vi "JLConfig Parse.vi"(0 "Config File Path":path=path "C:/Automation/Configurations/JusticeLeague.ini", 11 "Error In":errorcluster) -> (4 "Pass/Fail?":bool, 6 "Report Text":string, 8 "JusticeLeague_config":T1, 10 "Calibrate":bool, 15 "Error Out":errorcluster)   [LabVIEW 2019]
uses:
  type defs/JLConfig.ctl
  <vilib>/Utility/config.llb/Read Key (String).vi
  <vilib>/Utility/config.llb/Read Key (Boolean).vi
  <vilib>/Utility/config.llb/Read Key (Double).vi
  <vilib>/Utility/config.llb/NI_LVConfig.lvlib
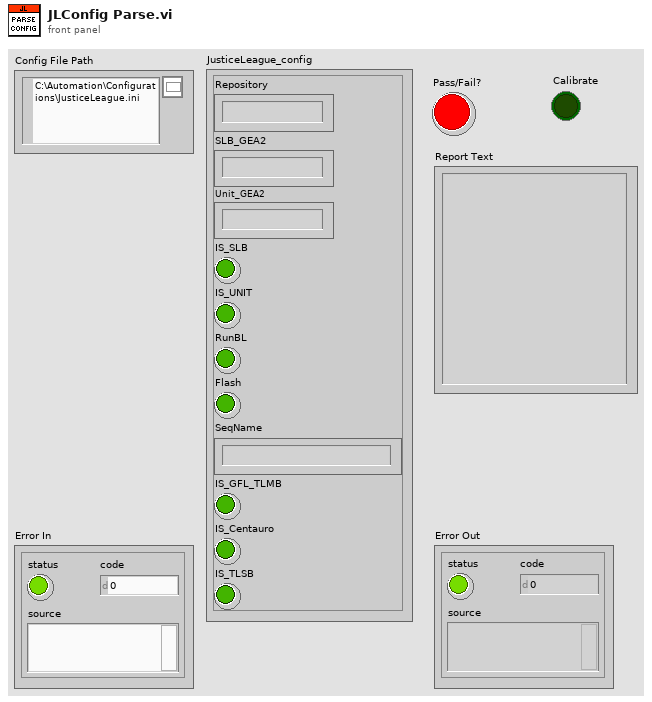
[diagram p1: front panel]
types:
  T1 = typedef "JLConfig.ctl" = cluster{"Repository":string, "SLB_GEA2":string, "Unit_GEA2":string, "IS_SLB":bool, "IS_UNIT":bool, "RunBL":bool, "Flash":bool, "SeqName":string, "IS_GFL_TLMB":bool, "IS_Centauro":bool, "IS_TLSB":bool}
  T2 = cluster{"Calibrate?":bool, "Scalling In ":cluster{"Raw Low ":dbl, "Raw High":dbl, "Actual Low":dbl, "Actual High":dbl}}
  T3 = typedef "NI_LVConfig.lvlib/Config Data RefNum.ctl" = refnum<k1>
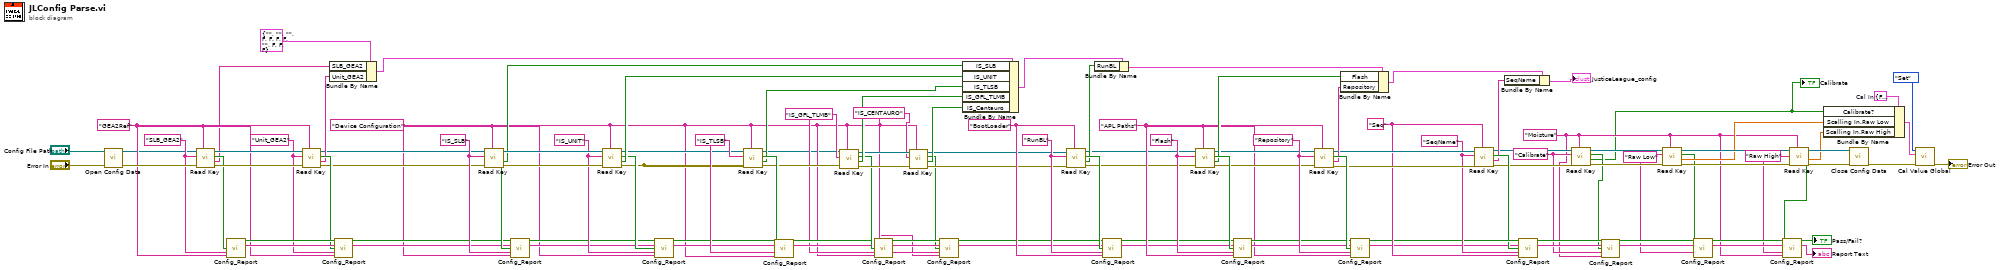
[diagram p0: block diagram]
diagram:
  w14 = "IS_TLSB" ("key")
  w5 = "IS_CENTAURO" ("key")
  w6 = "IS_GFL_TLMB" ("key")
  w34 = "Raw High" ("key")
  w35 = "Raw Low" ("key")
  w51 = T2 {"Calibrate?"=FALSE, "Scalling In "={"Raw Low "=1531.0, "Raw High"=6859.0, "Actual Low"=1.0, "Actual High"=4.9}}  # Cal In
  w33 = "Moisture" ("key")
  w39 = "Calibrate" ("key")
  w65 = "BootLoader" ("key")
  w70 = "RunBL" ("key")
  w83 = "SeqName" ("key")
  w82 = "Seq" ("section")
  w92 = "Repository" ("key")
  w31 = "IS_UNIT" ("key")
  w104 = "Flash" ("key")
  w79 = "APL Paths" ("section")
  w106 = "IS_SLB" ("key")
  w3 = "Device Configuration" ("section")
  w108 = "Unit_GEA2" ("key")
  w113 = "SLB_GEA2" ("key")
  w103 = "GEA2Ref" ("section")
  n1 = call <vilib>:"Open Config Data.vi"("error in (no error)"="Error In", "configuration file path"="Config File Path") -> ("error out"=w116:errorcluster, "refnum"=w86:T3)  [unwired: 7 in, 1 out]
  n2 = call-poly <vilib>:"Read Key.vi"("section"=w103, "error in (no error)"=w116, "key"=w113, "refnum"=w86) -> ("error out"=w117:errorcluster, "value"=w102:string, "found?"=w112:bool, "refnum out"=w118:T3)  [unwired: 4 in]
  n3 = call "Config_Report.vi"("Found?"=w112, "Key"=w113, "Section"=w103) -> ("Pass/Fail"=w111:bool, "Report Text"=w110:string)  [unwired: 11 in]
  n4 = call-poly <vilib>:"Read Key.vi"("section"=w103, "error in (no error)"=w117, "key"=w108, "refnum"=w118) -> ("error out"=w73:errorcluster, "value"=w101:string, "found?"=w109:bool, "refnum out"=w72:T3)  [unwired: 4 in]
  n5 = Bundle By Name(cluster=T1 {"Repository"="", "SLB_GEA2"="", "Unit_GEA2"="", "IS_SLB"=FALSE, "IS_UNIT"=FALSE, "RunBL"=FALSE, "Flash"=FALSE, "SeqName"="", "IS_GFL_TLMB"=FALSE, "IS_Centauro"=FALSE, "IS_TLSB"=FALSE} ("VALEW_config"), "SLB_GEA2"=w102, "Unit_GEA2"=w101) -> (w97:T1)
  n6 = call "Config_Report.vi"("Previous Pass/Fail"=w111, "Previous Report Text"=w110, "Found?"=w109, "Key"=w108, "Section"=w103) -> ("Pass/Fail"=w74:bool, "Report Text"=w75:string)  [unwired: 9 in]
  n7 = call-poly <vilib>:"Read Key.vi"("section"=w3, "error in (no error)"=w73, "key"=w106, "refnum"=w72) -> ("error out"=w99:errorcluster, "value"=w95:bool, "found?"=w107:bool, "refnum out"=w100:T3)  [unwired: 4 in]
  n8 = call "Config_Report.vi"("Previous Pass/Fail"=w74, "Previous Report Text"=w75, "Found?"=w107, "Key"=w106, "Section"=w3) -> ("Pass/Fail"=w29:bool, "Report Text"=w28:string)  [unwired: 9 in]
  n9 = call-poly <vilib>:"Read Key.vi"("section"=w3, "error in (no error)"=w99, "key"=w31, "refnum"=w100) -> ("error out"=w11:errorcluster, "value"=w96:bool, "found?"=w30:bool, "refnum out"=w12:T3)  [unwired: 4 in]
  n10 = call "Config_Report.vi"("Previous Pass/Fail"=w29, "Previous Report Text"=w28, "Found?"=w30, "Key"=w31, "Section"=w3) -> ("Pass/Fail"=w9:bool, "Report Text"=w10:string)  [unwired: 9 in]
  n11 = call-poly <vilib>:"Read Key.vi"("section"=w3, "error in (no error)"=w11, "key"=w14, "refnum"=w12) -> ("value"=w4:bool, "found?"=w13:bool, "refnum out"=w1:T3)  [unwired: 4 in, 1 out]
  n12 = call "Config_Report.vi"("Previous Pass/Fail"=w9, "Previous Report Text"=w10, "Found?"=w13, "Key"=w14, "Section"=w3) -> ("Pass/Fail"=w8:bool, "Report Text"=w7:string)  [unwired: 9 in]
  n13 = call-poly <vilib>:"Read Key.vi"("section"=w3, "error in (no error)"=w11, "key"=w6, "refnum"=w1) -> ("error out"=w19:errorcluster, "value"=w22:bool, "found?"=w16:bool, "refnum out"=w21:T3)  [unwired: 4 in]
  n14 = call "Config_Report.vi"("Previous Pass/Fail"=w8, "Previous Report Text"=w7, "Found?"=w16, "Key"=w6, "Section"=w3) -> ("Pass/Fail"=w26:bool, "Report Text"=w27:string)  [unwired: 9 in]
  n15 = call-poly <vilib>:"Read Key.vi"("section"=w3, "error in (no error)"=w19, "key"=w5, "refnum"=w21) -> ("error out"=w18:errorcluster, "value"=w23:bool, "found?"=w15:bool, "refnum out"=w20:T3)  [unwired: 4 in]
  n16 = call "Config_Report.vi"("Previous Pass/Fail"=w26, "Previous Report Text"=w27, "Found?"=w15, "Key"=w5, "Section"=w3) -> ("Pass/Fail"=w25:bool, "Report Text"=w24:string)  [unwired: 9 in]
  n17 = Bundle By Name(cluster=w97, "IS_SLB"=w95, "IS_UNIT"=w96, "IS_TLSB"=w4, "IS_GFL_TLMB"=w22, "IS_Centauro"=w23) -> (w71:T1)
  n18 = call-poly <vilib>:"Read Key.vi"("section"=w65, "error in (no error)"=w18, "key"=w70, "refnum"=w20) -> ("error out"=w17:errorcluster, "value"=w68:bool, "found?"=w69:bool, "refnum out"=w63:T3)  [unwired: 4 in]
  n19 = Bundle By Name(cluster=w71, "RunBL"=w68) -> (w64:T1)
  n20 = call "Config_Report.vi"("Previous Pass/Fail"=w25, "Previous Report Text"=w24, "Found?"=w69, "Key"=w70, "Section"=w65) -> ("Pass/Fail"=w67:bool, "Report Text"=w66:string)  [unwired: 9 in]
  n21 = call-poly <vilib>:"Read Key.vi"("section"=w79, "error in (no error)"=w17, "key"=w104, "refnum"=w63) -> ("error out"=w88:errorcluster, "value"=w94:bool, "found?"=w105:bool, "refnum out"=w89:T3)  [unwired: 4 in]
  n22 = call "Config_Report.vi"("Previous Pass/Fail"=w67, "Previous Report Text"=w66, "Found?"=w105, "Key"=w104, "Section"=w79) -> ("Pass/Fail"=w91:bool, "Report Text"=w90:string)  [unwired: 9 in]
  n23 = call-poly <vilib>:"Read Key.vi"("section"=w79, "error in (no error)"=w88, "key"=w92, "refnum"=w89) -> ("error out"=w85:errorcluster, "value"=w87:string, "found?"=w93:bool, "refnum out"=w84:T3)  [unwired: 4 in]
  n24 = Bundle By Name(cluster=w64, "Flash"=w94, "Repository"=w87) -> (w78:T1)
  n25 = call "Config_Report.vi"("Previous Pass/Fail"=w91, "Previous Report Text"=w90, "Found?"=w93, "Key"=w92, "Section"=w79) -> ("Pass/Fail"=w81:bool, "Report Text"=w76:string)  [unwired: 9 in]
  n26 = call-poly <vilib>:"Read Key.vi"("section"=w82, "error in (no error)"=w85, "key"=w83, "refnum"=w84) -> ("error out"=w62:errorcluster, "value"=w77:string, "found?"=w80:bool, "refnum out"=w61:T3)  [unwired: 4 in]
  n27 = Bundle By Name(cluster=w78, "SeqName"=w77) -> (→"JusticeLeague_config":T1)
  n28 = call "Config_Report.vi"("Previous Pass/Fail"=w81, "Previous Report Text"=w76, "Found?"=w80, "Key"=w83, "Section"=w82) -> ("Pass/Fail"=w47:bool, "Report Text"=w42:string)  [unwired: 9 in]
  n29 = call-poly <vilib>:"Read Key.vi"("section"=w33, "error in (no error)"=w62, "key"=w39, "refnum"=w61) -> ("error out"=w59:errorcluster, "value"=w32:bool, "found?"=w38:bool, "refnum out"=w60:T3)  [unwired: 4 in]
  "Calibrate" <- w32
  n30 = call "Config_Report.vi"("Previous Pass/Fail"=w47, "Previous Report Text"=w42, "Found?"=w38, "Key"=w39, "Section"=w33) -> ("Pass/Fail"=w46:bool, "Report Text"=w41:string)  [unwired: 9 in]
  n31 = call-poly <vilib>:"Read Key.vi"("section"=w33, "error in (no error)"=w59, "key"=w35, "refnum"=w60) -> ("error out"=w57:errorcluster, "value"=w50:dbl, "found?"=w37:bool, "refnum out"=w58:T3)  [unwired: 4 in]
  n32 = call "Config_Report.vi"("Previous Pass/Fail"=w46, "Previous Report Text"=w41, "Found?"=w37, "Key"=w35) -> ("Pass/Fail"=w45:bool, "Report Text"=w40:string)  [unwired: 10 in]
  n33 = call-poly <vilib>:"Read Key.vi"("section"=w33, "error in (no error)"=w57, "key"=w34, "refnum"=w58) -> ("error out"=w56:errorcluster, "value"=w49:dbl, "found?"=w36:bool, "refnum out"=w55:T3)  [unwired: 4 in]
  n34 = call "Config_Report.vi"("Previous Pass/Fail"=w45, "Previous Report Text"=w40, "Found?"=w36, "Key"=w34, "Section"=w33) -> ("Pass/Fail"=→"Pass/Fail?":bool, "Report Text"=→"Report Text":string)  [unwired: 9 in]
  n35 = Bundle By Name(cluster=w51, "Calibrate?"=w32, "Scalling In.Raw Low"=w50, "Scalling In.Raw High"=w49) -> (w48:T2)
  n36 = call <vilib>:"Close Config Data.vi"("error in (no error)"=w56, "refnum"=w55) -> ("error out"=w53:errorcluster)  [unwired: 8 in, 1 out]
  n37 = call "Cal Value Global.vi"("error in (no error)"=w53, "Cal In"=w48, "Action"=enum16{"Set", "Get "}."Set") -> ("error out"=→"Error Out":errorcluster)  [unwired: 7 in, 1 out]
